vi "PacketLost(SubVI).vi"(11 "PacketCounter":u32) -> (1 "Lost":bool, 2 "x-y":i32, 3 "CountLostPack out":u32)   [LabVIEW 2017]
panel:
  out "PacketNumberLast":u32
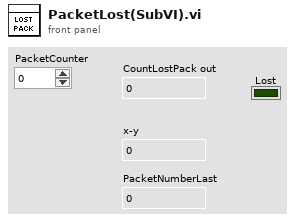
[diagram p1: front panel]
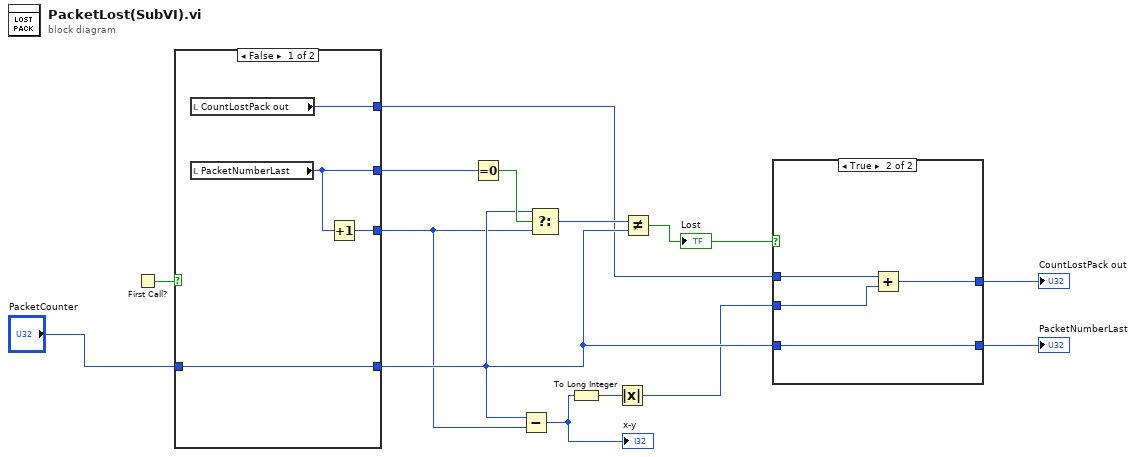
[diagram p0: block diagram]
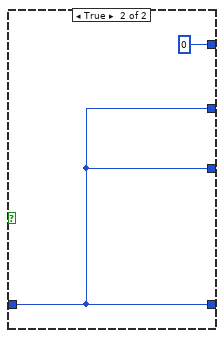
[diagram p2: hidden frame]
diagram:
  n1 = First Call?() -> (First Call?: T/F=w9:bool)
  n2 = case shown="False" w9 {
    tunnel: [w15 w19] -> w8
    tunnel: [w18 w19] -> w7
    tunnel: "PacketCounter" -> [w18 w19]
    tunnel: [w17 u32 0 ("CountLostPack out")] -> w6
    tunnel: [w16 w19] -> w2
    frame False {
      n3 = local read "CountLostPack out"() -> (w17:u32)
      n4 = local read "PacketNumberLast"() -> (w15:u32)
      n5 = Increment(x=w15) -> (x+1=w16:u32)
    }
    frame True {
    }
  }
  n6 = Equal To 0?(x=w8) -> (x = 0?=w11:bool)
  n7 = Subtract(x=w7, y=w2) -> (x-y=w5:u32)
  "x-y" <- w5
  n8 = Select(t=w7, s=w11, f=w2) -> (s? t:f=w12:u32)
  n9 = To Long Integer(number=w5) -> (32bit integer=w4:i32)
  n10 = Absolute Value(x=w4) -> (abs(x)=w3:i32)
  n11 = Not Equal?(x=w12, y=w7) -> (x != y?=w13:bool)
  "Lost" <- w13
  n12 = case shown="True" w13 {
    tunnel: w6 -> [w22 w25]
    tunnel: [w22 w23] -> w14
    tunnel: w7 -> [w21 w26]
    tunnel: [w21 w26] -> w10
    tunnel: w3 -> [_ w24]
    frame False {
    }
    frame True {
      n13 = Add(x=w25, y=w24) -> (x+y=w23:u32)
    }
  }
  "CountLostPack out" <- w14
  "PacketNumberLast" <- w10
